vi "Main.vi"(8 "error in":errorcluster, 11 "DB File Path in":path=path "C:/Users/OneEd/OneDrive/Desktop/MicroPort Job/Component Tracing/MPCT.db") -> (0 "error out":errorcluster)   [LabVIEW 2021]
uses:
  SQL-LV Table File Paths.ctl
  SQL-LV Table Control Paths.ctl
  SQL-LV Table VI Paths.ctl
  edt.lib/sqlite.lib/SQLite Foreign Key.ctl
  edt.lib/sqlite.lib/SQLite Reaction Type.ctl
  SQL-LV View File Paths.ctl
  SQL-LV View Control Paths.ctl
  SQL-LV View VI Paths.ctl
  <vilib>/drjdpowell/SQLite Library/SQL Connection/Connection.lvclass
  edt.lib/sqlite.lib/EDT SQLite+.lvlib
panel:
  out "Array 2":T1[](array[typedef])
  in  "View Folder":path=path "C:/Users/OneEd/OneDrive/Desktop/MicroPort Job/Component Tracing/src/SQL Function/View"
  out "Slide":dbl(slide) scale=0.0..1.0
  out "Foreign Key List":T4[](array[typedef])
  out "Array":T6[](array[typedef])
  in  "Table Folder":path=path "C:/Users/OneEd/OneDrive/Desktop/MicroPort Job/Component Tracing/src/SQL Function/Table"
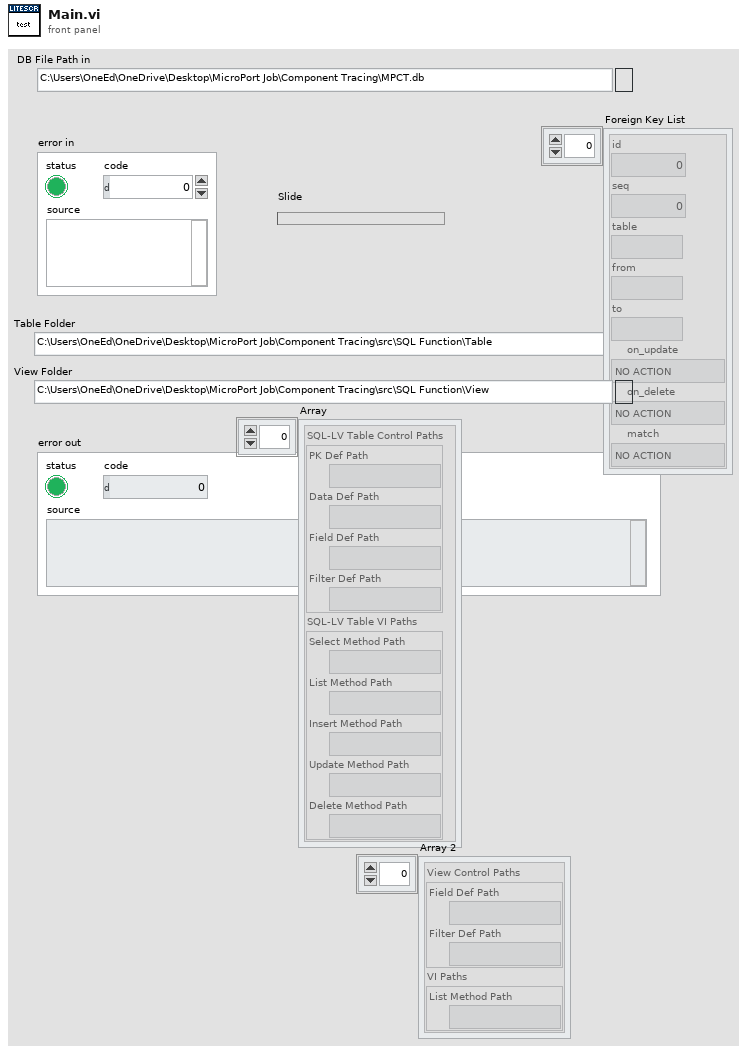
[diagram p1: front panel]
types:
  T1 = typedef "SQL-LV View File Paths.ctl" = cluster{"View Control Paths":T2, "VI Paths":T3}
  T2 = typedef "SQL-LV View Control Paths.ctl" = cluster{"Field Def Path":path, "Filter Def Path":path}
  T3 = typedef "SQL-LV View VI Paths.ctl" = cluster{"List Method Path":path}
  T4 = typedef "EDT SQLite+.lvlib/SQLite Foreign Key.ctl" = cluster{"id":i64, "seq":i64, "table":string, "from":string, "to":string, "on_update":T5, "on_delete":T5, "match":T5}
  T5 = typedef "EDT SQLite+.lvlib/SQLite Reaction Type.ctl" = enum16{"NO ACTION", "SET NULL", "SET DEFAULT", "CASCADE", "RESTRICT", "NONE"}
  T6 = typedef "SQL-LV Table File Paths.ctl" = cluster{"SQL-LV Table Control Paths":T7, "SQL-LV Table VI Paths":T8}
  T7 = typedef "SQL-LV Table Control Paths.ctl" = cluster{"PK Def Path":path, "Data Def Path":path, "Field Def Path":path, "Filter Def Path":path}
  T8 = typedef "SQL-LV Table VI Paths.ctl" = cluster{"Select Method Path":path, "List Method Path":path, "Insert Method Path":path, "Update Method Path":path, "Delete Method Path":path}
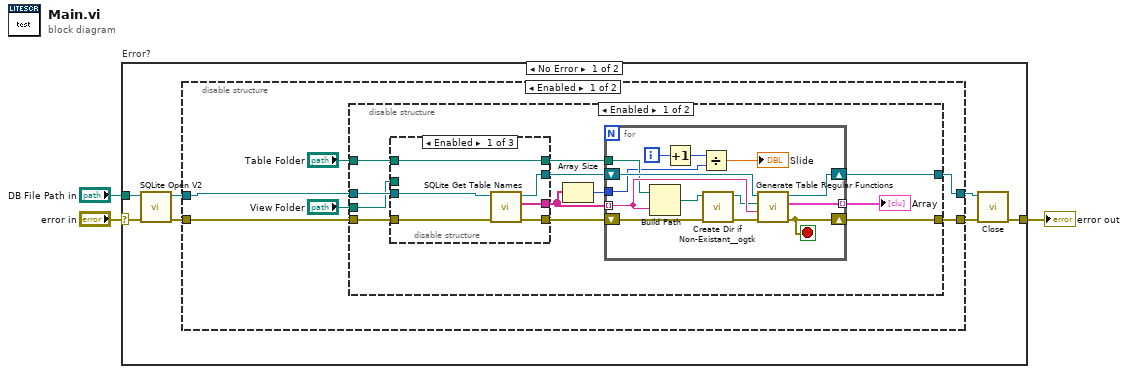
[diagram p0: block diagram]
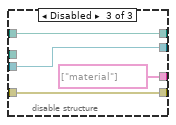
[diagram p3: hidden frame]
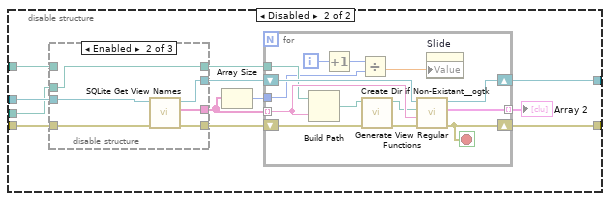
[diagram p4: hidden frame]
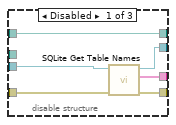
[diagram p5: hidden frame]
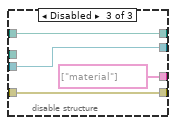
[diagram p6: hidden frame]
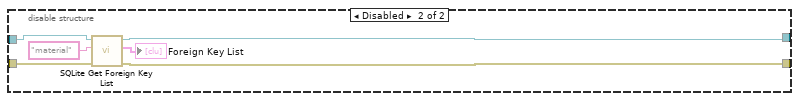
[diagram p7: hidden frame]
diagram:
  n1 = case "Error?" shown="No Error" "error in" {
    selector: "error in" -> [w10 w101]
    tunnel: "DB File Path in" -> [w9 _]
    tunnel: [w4 w101] -> w2
    frame No Error {
      n2 = call "SQLite Open V2.vi"("error in"=w10, "File Path"=w9) -> ("error out"=w8:errorcluster, "SQLite Connection"=w7:refnum<class "Connection.lvclass">)  [unwired: 7 in, 1 out]
      n3 = disable-structure shown="Enabled" {
        disable-tunnel: w8 -> [w13 w99]
        disable-tunnel: w7 -> [w14 w100]
        disable-tunnel: [w15 w97] -> w6
        disable-tunnel: [w16 w98] -> w5
        frame Enabled {
          n4 = disable-structure shown="Enabled" {
            disable-tunnel: [w28 w64] -> w16
            disable-tunnel: [w27 w63] -> w15
            disable-tunnel: w14 -> [w26 w62]
            disable-tunnel: w13 -> [w24 w60]
            disable-tunnel: "Table Folder" -> [w19 w55]
            disable-tunnel: "View Folder" -> [w18 w54]
            frame Enabled {
              n5 = disable-structure shown="Enabled" {
                disable-tunnel: w26 -> [w34 _ w38]
                disable-tunnel: [w33 _ w38] -> w25
                disable-tunnel: w24 -> [w32 _ w37]
                disable-tunnel: [w31 _ w37] -> w23
                disable-tunnel: [w30 _ string[] ["material"] ("Table Names")] -> w22
                disable-tunnel: [w29 _ w35] -> w20
                disable-tunnel: w19 -> [w29 _ w35]
                disable-tunnel: w18 -> [_ _ _]
                frame Enabled {
                  n6 = call "SQLite Get Table Names.vi"("error in"=w32, "SQLite Connection"=w34) -> ("error out"=w31:errorcluster, "Table Names"=w30:string[], "Dup SQLite Connection"=w33:refnum<class "Connection.lvclass">)  [unwired: 7 in]
                }
                frame Disabled {
                }
                frame Disabled {
                }
              }
              n7 = Array Size(array=w22) -> (size(s)=w21:i32)
              n8 = for {
                tunnel: w20 -> [w47]
                shift-right: [w49] -> w28
                shift-left: w23 -> [w44]
                shift-right: [w52] -> w27
                shift-left: w25 -> [w51]
                tunnel: w22 -> [w48] mode=indexing
                tunnel: [w50] -> w17 mode=indexing
                tunnel: w21 -> [w40]
                i -> [w42]
                stop <- w49 stop-if-true
                n9 = Build Path(base path=w47, name or relative path=w48) -> (appended path=w46:path)
                n10 = Increment(x=w42) -> (x+1=w41:i32)
                n11 = Divide(x=w41, y=w40) -> (x/y=→"Slide":dbl)
                n12 = call <userlib>:"Create Dir if Non-Existant__ogtk.vi"("error in (no error)"=w44, "Directory Path"=w46) -> ("error out"=w43:errorcluster, "dup Directory Path"=w45:path)  [unwired: 7 in, 1 out]
                n13 = call "Generate Table Regular Functions.vi"("Error in"=w43, "Table Name"=w48, "Folder to Saved File"=w45, "Connection in"=w51) -> ("Error out"=w49:errorcluster, "SQL-LV File Paths"=w50:T6, "Connection out"=w52:refnum<class "Connection.lvclass">)  [unwired: 5 in]
              }
              "Array" <- w17
            }
            frame Disabled {
              n14 = disable-structure shown="Enabled" {
                disable-tunnel: w62 -> [w70 w76 w80]
                disable-tunnel: [w69 w75 w80] -> w61
                disable-tunnel: w60 -> [w68 w74 w79]
                disable-tunnel: [w67 w73 w79] -> w59
                disable-tunnel: [w66 w72 string[] ["material"] ("Table Names")] -> w58
                disable-tunnel: [w65 w71 w77] -> w56
                disable-tunnel: w55 -> [w65 _ w77]
                disable-tunnel: w54 -> [_ w71 _]
                frame Disabled {
                  n15 = call "SQLite Get Table Names.vi"("error in"=w68, "SQLite Connection"=w70) -> ("error out"=w67:errorcluster, "Table Names"=w66:string[], "Dup SQLite Connection"=w69:refnum<class "Connection.lvclass">)  [unwired: 7 in]
                }
                frame Enabled {
                  n16 = call "SQLite Get View Names.vi"("error in"=w74, "SQLite Connection"=w76) -> ("error out"=w73:errorcluster, "View Names"=w72:string[], "Dup SQLite Connection"=w75:refnum<class "Connection.lvclass">)  [unwired: 7 in]
                }
                frame Disabled {
                }
              }
              n17 = Array Size(array=w58) -> (size(s)=w57:i32)
              n18 = for {
                tunnel: w56 -> [w89]
                shift-right: [w91] -> w64
                shift-left: w59 -> [w86]
                shift-right: [w94] -> w63
                shift-left: w61 -> [w93]
                tunnel: w58 -> [w90] mode=indexing
                tunnel: [w92] -> w53 mode=indexing
                tunnel: w57 -> [w82]
                i -> [w84]
                stop <- w91 stop-if-true
                n19 = Build Path(base path=w89, name or relative path=w90) -> (appended path=w88:path)
                n20 = Increment(x=w84) -> (x+1=w83:i32)
                n21 = Divide(x=w83, y=w82) -> (x/y=w81:dbl)
                n22 = call <userlib>:"Create Dir if Non-Existant__ogtk.vi"("error in (no error)"=w86, "Directory Path"=w88) -> ("error out"=w85:errorcluster, "dup Directory Path"=w87:path)  [unwired: 7 in, 1 out]
                n23 = call "Generate View Regular Functions.vi"("Error in"=w85, "Table Name"=w90, "Folder to Saved File"=w87, "Connection in"=w93) -> ("Error out"=w91:errorcluster, "SQL-LV File Paths"=w92:T1, "Connection out"=w94:refnum<class "Connection.lvclass">)  [unwired: 5 in]
                n24 = property on="Slide" class="Slide (strict)"("Value"=w81) -> ()  [unwired: 2 in, 2 out]
              }
              "Array 2" <- w53
            }
          }
        }
        frame Disabled {
          n25 = call "SQLite Get Foreign Key List.vi"("error in"=w99, "Table Name"="material", "SQLite Connection"=w100) -> ("error out"=w98:errorcluster, "Foreign Key List"=→"Foreign Key List":T4[], "Dup SQLite Connection"=w97:refnum<class "Connection.lvclass">)  [unwired: 6 in]
        }
      }
      n26 = call-dynamic "Close.vi"("error in (no error)"=w5, "SQLite Connection in"=w6) -> ("error out"=w4:errorcluster)  [unwired: 9 in]
    }
    frame Error {
    }
  }
  "error out" <- w2
